vi "Error.vi"() -> ()   [LabVIEW 2019]
panel:
  out "Compensated 2 PLCs":dbl[](array[numeric])=[8.118001821194379e-06, 3.028394010146989e-06, -1.1425160653180158e-05, -1.4517135469196977e-05, -4.108357520226165e-06] format="%#_6p"
  in  "Shorted 2 PLCs":dbl[](array[numeric])=[-6.648192609520545e-06, -2.6579412172609335e-06, 5.730660716698524e-06, 9.480335334891014e-06, -2.6031729589807576e-07] format="%#_7p"
  in  "Automated Measurements 2 PLCs":dbl[](array[numeric])=[3.4836450894493014, 3.4851235250583956, 3.4816668463890865, 3.4843693300881156, 3.4864364998877293] format="%#_7p"
  in  "Manual 7.5 digit":dbl[](array[numeric])=[3.483646559258513, 3.4851238955111885, 3.48166115188915, 3.4843642932879813, 3.486432131212913] format="%#_7p"
  out "Error 2 PLCs":dbl[](array[numeric])=[1.4698092116738337e-06, 3.704527928860557e-07, -5.694499936481634e-06, -5.036800134305963e-06, -4.368674816124241e-06] format="%#_6p"
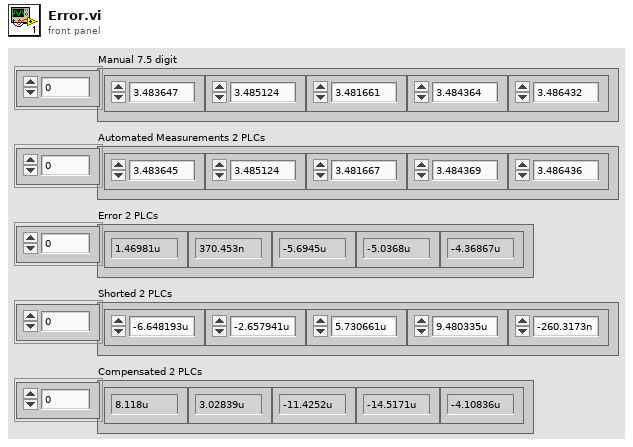
[diagram p1: front panel]
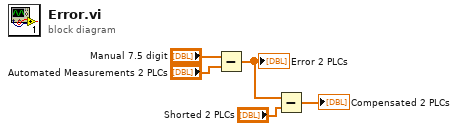
[diagram p0: block diagram]
diagram:
  n1 = Subtract(x="Manual 7.5 digit", y="Automated Measurements 2 PLCs") -> (x-y=w3:dbl[])
  "Error 2 PLCs" <- w3
  n2 = Subtract(x=w3, y="Shorted 2 PLCs") -> (x-y=→"Compensated 2 PLCs":dbl[])
